vi "Joystick axes.vi"(11 "Axes":dbl[](array[numeric])) -> (0 "Throttle":dbl, 1 "Z":dbl, 2 "X":dbl, 3 "Y":dbl)   [LabVIEW 2015]
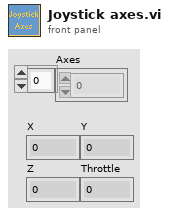
[diagram p1: front panel]
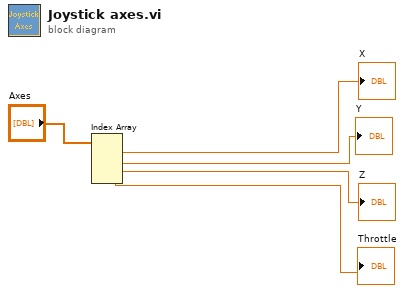
[diagram p0: block diagram]
diagram:
  n1 = Index Array(array="Axes") -> (element #1=→"X":dbl, element #2=→"Y":dbl, element #3=→"Z":dbl, element #4=→"Throttle":dbl)  [unwired: 4 in]
